vi "Get Parameter.vi"(8 "error in (no error)":errorcluster, 11 "result in":refnum<class "result.lvclass">) -> (0 "error out":errorcluster, 2 "Data":variant, 3 "result out":refnum<class "result.lvclass">)   [LabVIEW 2015, in "result.lvclass"]
uses:
  result.lvclass
  result.lvclass/result.ctl
  <vilib>/addons/lv-msgpack/MsgPack Deserializer/MsgPackDeserializer.lvclass
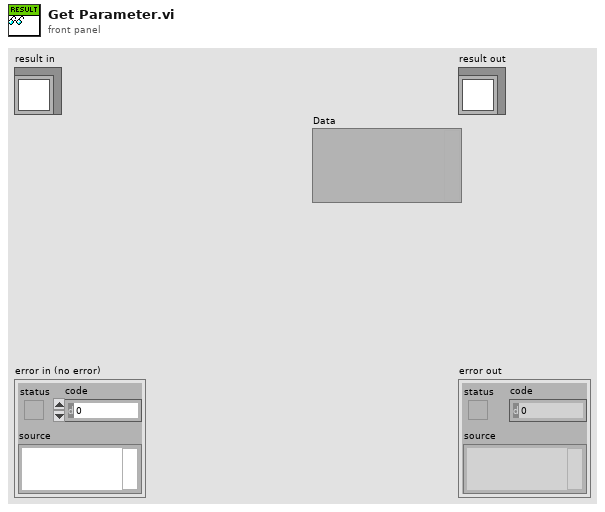
[diagram p1: front panel]
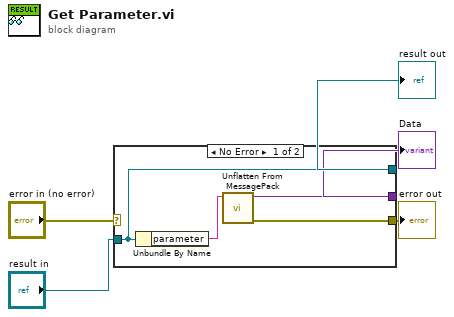
[diagram p0: block diagram]
diagram:
  n1 = case shown="No Error" "error in (no error)" {
    selector: "error in (no error)" -> [_ w10]
    tunnel: [w8 w10] -> w4
    tunnel: [w9 w11] -> w2
    tunnel: "result in" -> [w9 w11]
    tunnel: [w6 _] -> w1
    frame No Error {
      n2 = Unbundle By Name(w9) -> ("parameter"=w7:string)
      n3 = call <vilib>:"Unflatten From MessagePack.vi"("MsgPack Data"=w7) -> ("error IO"=w8:errorcluster, "Data"=w6:variant)  [unwired: 8 in, 1 out]
    }
    frame Error {
    }
  }
  "error out" <- w4
  "result out" <- w2
  "Data" <- w1
